vi "Disable Log.vi"(8 "error in (no error)":errorcluster, 9 "Stop Trigger Time":timestamp, 11 "Waveform Log in":refnum<class "Waveform Log.lvclass">) -> (0 "error out":errorcluster, 3 "Waveform Log out":refnum<class "Waveform Log.lvclass">)   [LabVIEW 2012, in "Waveform Data Logger Engine.lvlib" / "Waveform Log.lvclass"]
uses:
  Waveform Log.lvclass
  Waveform Log.lvclass/Waveform Log.ctl
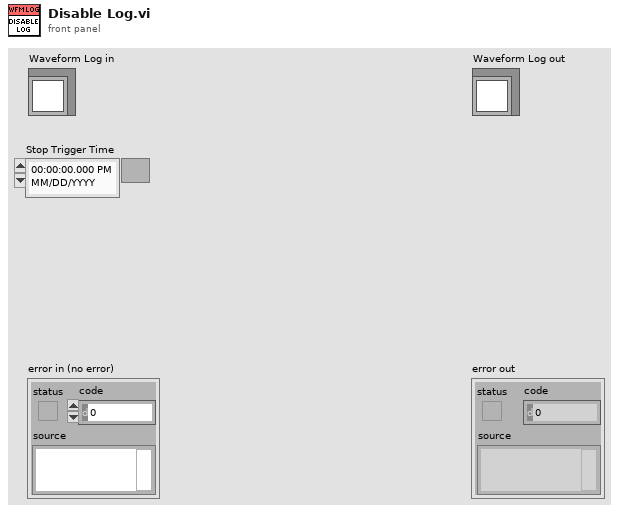
[diagram p1: front panel]
types:
  T1 = typedef "Waveform Data Logger Engine.lvlib/Waveform Log.lvclass/Log Instance.ctl" = cluster{"Segmented Log":refnum<data-value>, "Log Waveforms":T2[], "Log Start":timestamp, "Log Stop":timestamp, "Start Trigger Time":timestamp, "Stop Trigger Time":timestamp, "Time of Last Write":timestamp, "Timeout":dbl, "Stop cmd received":bool}
  T2 = typedef "Waveform Data Logger Engine.lvlib/Waveform Log.lvclass/Log Instance Waveform.ctl" = cluster{"Wfm Info":T3, "Count / Instance":i32, "Previous Segment":u64, "Wfm Complete?":bool, "Last Sample Logged":timestamp, "Data Logged":bool, "Log segmented":bool}
  T3 = typedef "Waveform Data Logger Engine.lvlib/Waveform Log.lvclass/Waveform Information.ctl" = cluster{"Name":string, "Wfm Data Type":T4, "Decimation":u32}
  T4 = typedef "Waveform Data Logger Engine.lvlib/Waveform Log.lvclass/Waveform Data Type.ctl" = enum16{"Double", "ComplexDouble"}
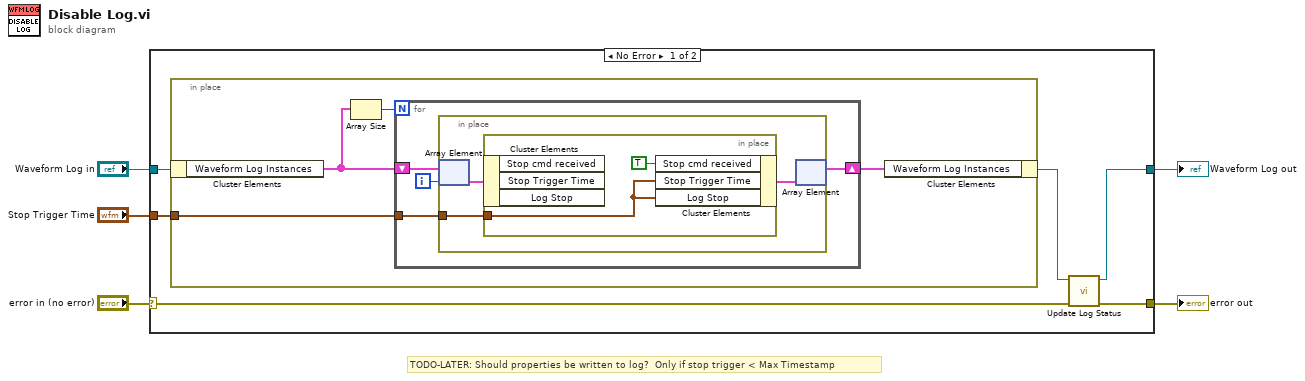
[diagram p0: block diagram]
diagram:
  # "TODO-LATER: Should properties be written to log?  Only if stop trigger < Max Timestamp"
  n1 = case shown="No Error" "error in (no error)" {
    selector: "error in (no error)" -> [w9 w26]
    tunnel: [w8 w26] -> w4
    tunnel: [w6 w25] -> w2
    tunnel: "Waveform Log in" -> [w11 w25]
    tunnel: "Stop Trigger Time" -> [w10 _]
    frame No Error {
      n2 = in-place {
        in-place-border: w10 -> [w14]
        n3 = in-place-cluster #1(w11) -> ("Waveform Log Instances"=w12:T1[])
        n4 = Array Size(array=w12) -> (size(s)=w13:i32)
        n5 = for {
          N: w13 -> [_]
          tunnel: w14 -> [w17]
          shift-right: [w18] -> w15
          shift-left: w12 -> [w19]
          i -> [w16]
          n6 = in-place {
            in-place-border: w17 -> [w22]
            n7 = in-place-array #2(w19, w16) -> (w21:T1)
            n8 = in-place {
              in-place-border: w22 -> [w23]
              n9 = in-place-cluster #3(w21) -> ()  [unwired: 3 out]
              n10 = in-place-cluster #3("Stop cmd received"=TRUE, "Stop Trigger Time"=w23, "Log Stop"=w23) -> (w20:T1)
            }
            n11 = in-place-array #2(w20) -> (w18:T1[])  [unwired: 1 out]
          }
        }
        n12 = in-place-cluster #1("Waveform Log Instances"=w15) -> (w7:refnum<class "Waveform Log.lvclass">)
      }
      n13 = call "Update Log Status.vi"("error in (no error)"=w9, "Waveform Log in"=w7) -> ("error out"=w8:errorcluster, "Waveform Log out"=w6:refnum<class "Waveform Log.lvclass">)  [unwired: 8 in]
    }
    frame Error {
    }
  }
  "error out" <- w4
  "Waveform Log out" <- w2
